vi "getVersionInfo.vi"(6 "DLLVersion":i8[](array[numeric]), 7 "Device":i32, 8 "error in (no error)":errorcluster, 9 "FirmwareVersion":i8[](array[numeric]), 10 "FPGAVersion":i8[](array[numeric]), 11 "SEDSpectrometer in":refnum<class "SEDSpectrometer.lvclass">) -> (0 "error out":errorcluster, 1 "FirmwareVersion":i8[](array[numeric]), 2 "FPGAVersion":i8[](array[numeric]), 3 "SEDSpectrometer out":refnum<class "SEDSpectrometer.lvclass">, 4 "DLLVersion":i8[](array[numeric]), 5 "Output Value":i32)   [LabVIEW 2016, in "SEDSpectrometer.lvclass"]
uses:
  SEDSpectrometer.lvclass
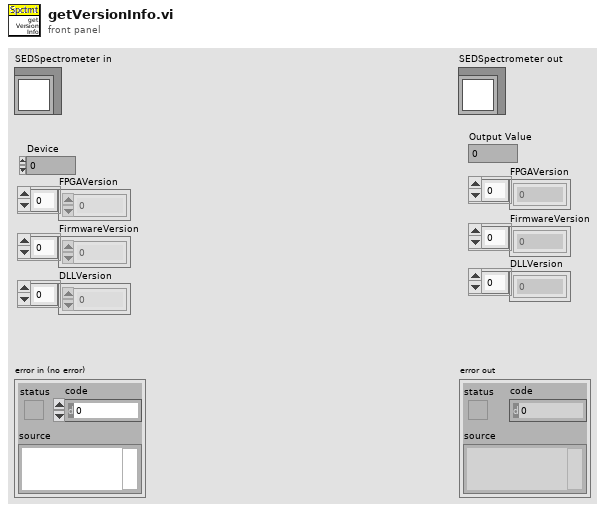
[diagram p1: front panel]
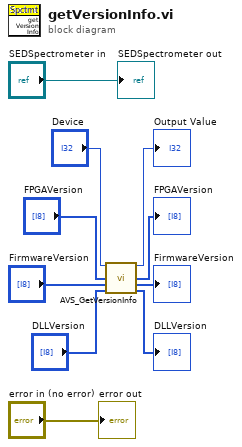
[diagram p0: block diagram]
diagram:
  n1 = call "AVS_GetVersionInfo.vi"("a_hDevice"="Device", "a_pFPGAVersion"="FPGAVersion", "a_pFirmwareVersion"="FirmwareVersion", "a_pDLLVersion"="DLLVersion") -> ("Output Value"=→"Output Value":i32, "a_pFPGAVersion"=→"FPGAVersion":i8[], "a_pFirmwareVersion"=→"FirmwareVersion":i8[], "a_pDLLVersion"=→"DLLVersion":i8[])  [unwired: 8 in]
  "error out" <- "error in (no error)"
  "SEDSpectrometer out" <- "SEDSpectrometer in"
